vi "Control Loop Que_NameArr.vi"(7 "Action Select":enum16{"Initial", "Add", "Release"}(ring)=enum."Release", 8 "error in (no error)":errorcluster, 11 "Control Loop In":T3) -> (0 "error out":errorcluster, 3 "Control Loop Q Out":refnum<queue>)   [LabVIEW 2019]
uses:
  Ctrl/Control Loop_Control.ctl
  Ctrl/Control Loop_Status.ctl
panel:
  in  "Name":string
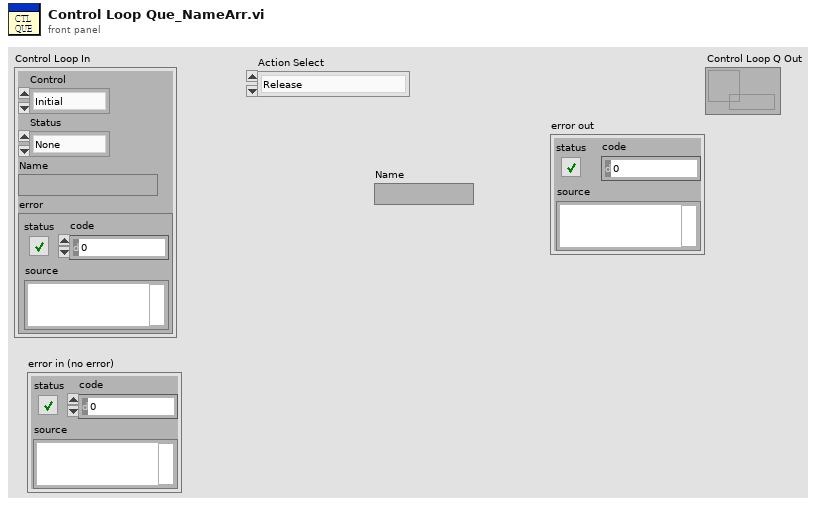
[diagram p1: front panel]
types:
  T1 = typedef "Control Loop_Control.ctl" = enum16{"Initial", "Standby Mode", "Run Mode", "Status", "Exit"}
  T2 = typedef "Control Loop_Status.ctl" = enum16{"None", "Next", "Error", "SafeDoor", "Exit"}
  T3 = cluster{"Control":T1, "Status":T2, "Name":string, "error":errorcluster}
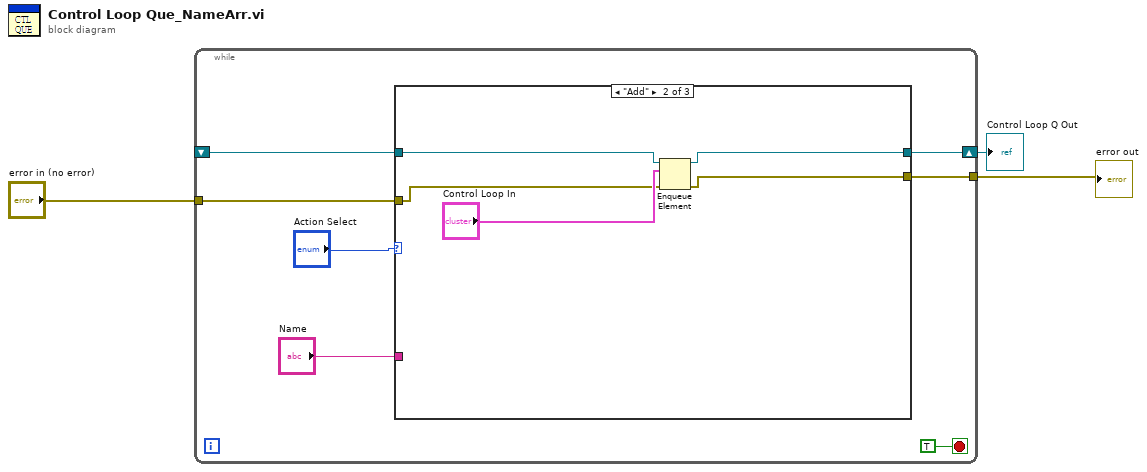
[diagram p0: block diagram]
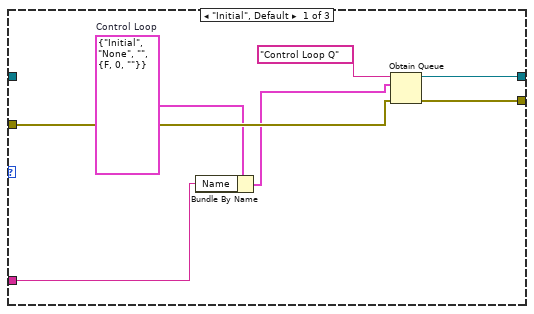
[diagram p2: hidden frame]
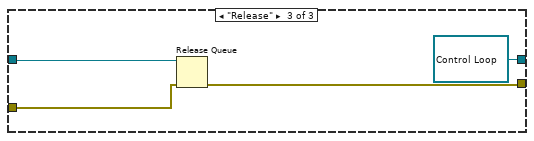
[diagram p3: hidden frame]
diagram:
  n1 = while {
    shift-right: [w10] -> w1
    shift-left: _ -> [w8]
    tunnel: "error in (no error)" -> [w7]
    tunnel: [w6] -> w2
    stop <- TRUE stop-if-true
    n2 = case shown="\"Add\"" "Action Select" {
      tunnel: [w17 w21 refnum<queue> refnum ("queue out")] -> w10
      tunnel: w8 -> [_ w22 w26]
      tunnel: w7 -> [w15 w18 w25]
      tunnel: [w14 w19 w24] -> w6
      tunnel: "Name" -> [w12 _ _]
      frame "Initial", Default {
        w13 = T3 {"Control"=enum."Initial", "Status"=enum."None", "Name"="", "error"={"status"=FALSE, "code"=0, "source"=""}}  # Control Loop
        n3 = Bundle By Name(cluster=w13, "Name"=w12) -> (w11:T3)
        n4 = Obtain Queue(name (unnamed)="Control Loop Q", element data type=w11, error in (no error)=w15) -> (queue out=w17:refnum<queue>, error out=w14:errorcluster)  [unwired: 2 in, 1 out]
      }
      frame "Add" {
        n5 = Enqueue Element(queue=w22, element="Control Loop In", error in (no error)=w18) -> (queue out=w21:refnum<queue>, error out=w19:errorcluster)  [unwired: 1 in, 1 out]
      }
      frame "Release" {
        n6 = Release Queue(queue=w26, error in (no error)=w25) -> (error out=w24:errorcluster)  [unwired: 1 in, 2 out]
      }
    }
  }
  "error out" <- w2
  "Control Loop Q Out" <- w1
